vi "initialise.vi"(8 "error in (no error)":errorcluster, 11 "TrajectoryCN090716SpiralScan in":refnum<class "TrajectoryCN090716SpiralScan.lvclass">) -> (0 "error out":errorcluster, 3 "TrajectoryCN090716SpiralScan out":refnum<class "TrajectoryCN090716SpiralScan.lvclass">)   [LabVIEW 2010, in "TrajectoryCN090716SpiralScan.lvclass"]
uses:
  TrajectoryCN090716SpiralScan.lvclass
  <vilib>/Native 3D Graph/xcontrol/3DPC_SurfacePlot.xctl
  TrajectoryDL091126GenericVoxel/TrajectoryDL091126GenericVoxel/TrajectoryDL091126GenericVoxel.lvclass
  common/enumerations/functional_global_action_enum.ctl
  common/enumerations/x_y_z_enumeration.ctl
  TrajectoryCN090716SpiralScan.lvclass/TrajectoryCN090716SpiralScan.ctl
panel:
  out "z signal":dbl[](graph)
  out "3D Graph":refnum<class "Base Datatype.lvclass">[](xcontrol)
  out "x signal":dbl[](graph)
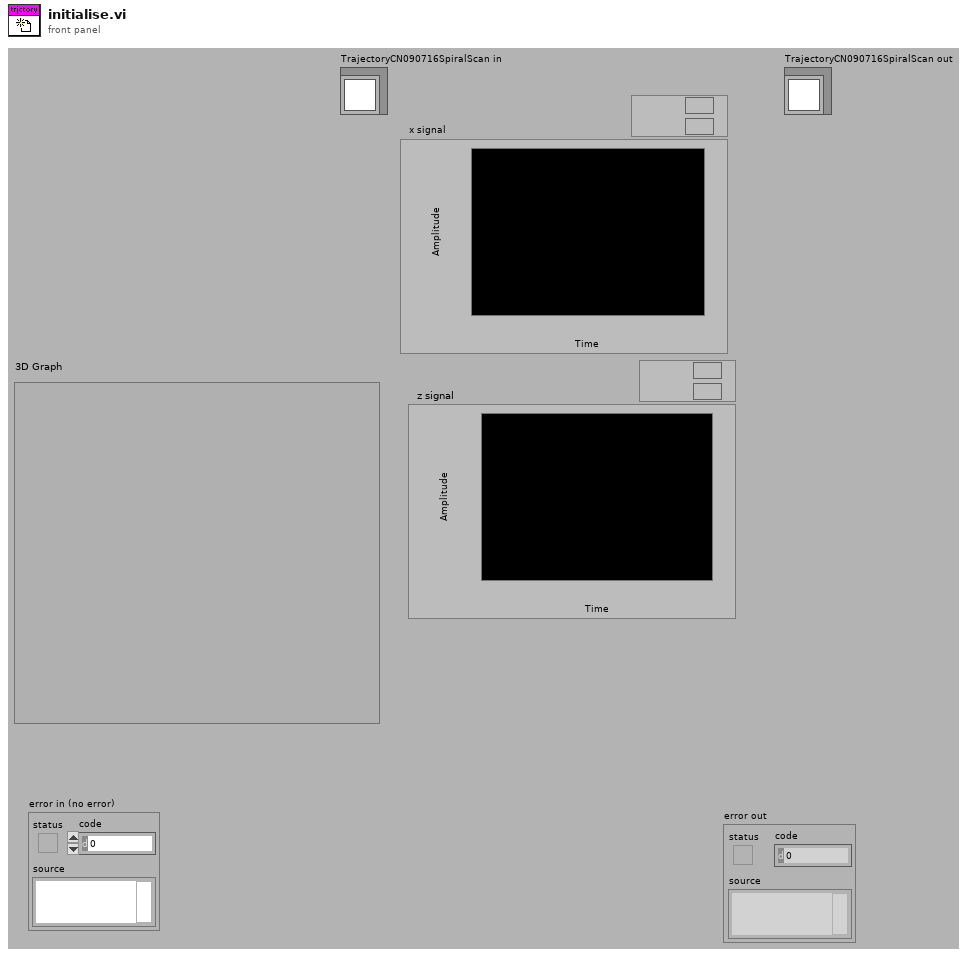
[diagram p1: front panel]
types:
  T1 = typedef "x_y_z_enumeration.ctl" = enum16{"x", "y", "z"}
  T2 = typedef "functional_global_action_enum.ctl" = enum16{"get", "set", "reset"}
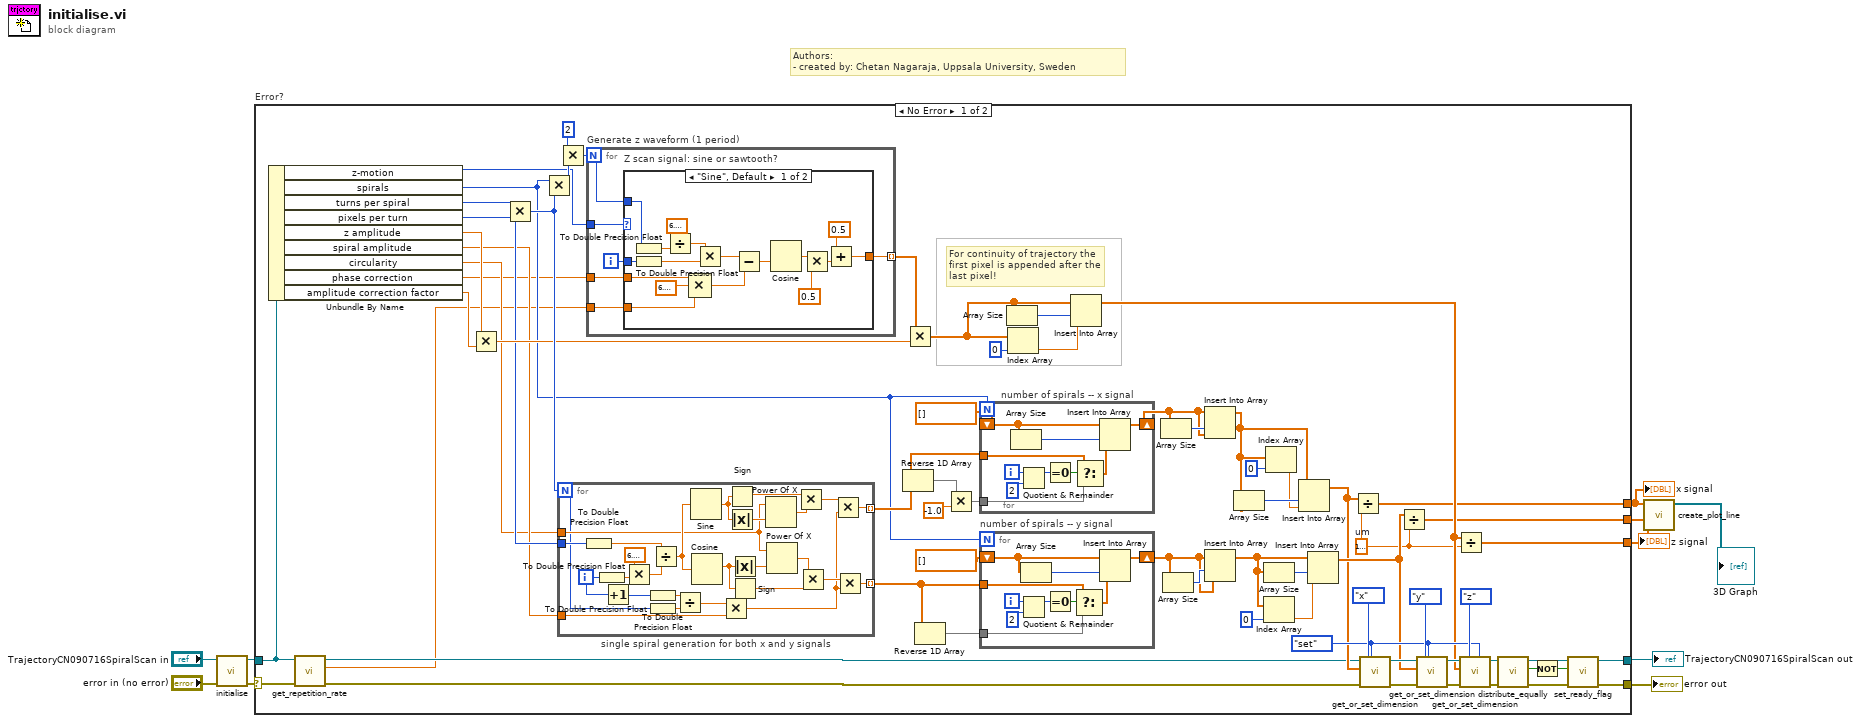
[diagram p0: block diagram]
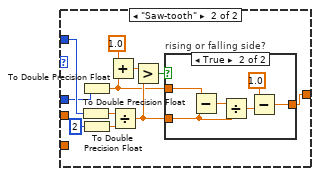
[diagram p2: hidden frame]
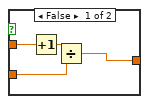
[diagram p3: hidden frame]
diagram:
  # "Authors: \n- created by: Chetan Nagaraja, Uppsala University, Sweden"
  n1 = call-parent "initialise.vi"("error in (no error)"="error in (no error)", "GenericTrajectory in"="TrajectoryCN090716SpiralScan in") -> ("error out"=w5:errorcluster, "GenericTrajectory out"=w6:refnum<class "TrajectoryCN090716SpiralScan.lvclass">)  [unwired: 8 out]
  n2 = case "Error?" shown="No Error" w5 {
    selector: w5 -> [w15 w169]
    tunnel: w6 -> [w13 w170]
    tunnel: [w33 w170] -> w10
    tunnel: [w30 w169] -> w9
    tunnel: [w39 _] -> w1
    tunnel: [w38 _] -> w3
    tunnel: [w29 _] -> w2
    frame No Error {
      w27 = dbl[unit] 1e-06  # um
      w70 = functional_global_action_enum."set" ("action")
      # "For continuity of trajectory the\nfirst pixel is appended after the \nlast pixel!"
      n3 = Unbundle By Name(w13) -> ("z-motion"=w22:enum16{"Sine", "Saw-tooth"}, "spirals"=w24:i32, "turns per spiral"=w23:i32, "pixels per turn"=w25:i32, "z amplitude"=w21:dbl[unit], "spiral amplitude"=w20:dbl[unit], "circularity"=w19:dbl, "phase correction"=w18:dbl[unit], "amplitude correction factor"=w17:dbl)
      n4 = call-dynamic "get_repetition_rate.vi"("error in (no error)"=w15, "GenericTrajectory in"=w13) -> ("error out"=w14:errorcluster, "repetition rate"=w11:dbl[unit], "GenericTrajectory out"=w12:refnum<class "TrajectoryCN090716SpiralScan.lvclass">)  [unwired: 7 in]
      n5 = Multiply(x=w21, y=w17) -> (x*y=w26:dbl[unit])
      n6 = Multiply(x=w23, y=w25) -> (x*y=w66:i32)
      n7 = Multiply(x=w24, y=w66) -> (x*y=w65:i32)
      n8 = Multiply(x=2, y=w65) -> (x*y=w59:i32)
      n9 = for "single spiral generation for both x and y signals" {
        N: w66 -> [w142]
        tunnel: w20 -> [w145]
        tunnel: [w156] -> w60 mode=indexing
        tunnel: [w155] -> w62 mode=indexing
        tunnel: w19 -> [w154]
        tunnel: w25 -> [w151]
        i -> [w146]
        n10 = To Double Precision Float(number=w151) -> (double precision float=w150:dbl)
        n11 = To Double Precision Float(number=w146) -> (double precision float=w152:dbl)
        n12 = Increment(x=w146) -> (x+1=w143:i32)
        n13 = Multiply(x=6.283185307179586, y=w152) -> (x*y=w153:dbl)
        n14 = To Double Precision Float(number=w143) -> (double precision float=w149:dbl)
        n15 = To Double Precision Float(number=w142) -> (double precision float=w148:dbl)
        n16 = Divide(x=w153, y=w150) -> (x/y=w160:dbl)
        n17 = Divide(x=w149, y=w148) -> (x/y=w147:dbl)
        n18 = Sine(x=w160) -> (sin(x)=w168:dbl)
        n19 = Cosine(x=w160) -> (cos(x)=w167:dbl)
        n20 = Multiply(x=w147, y=w145) -> (x*y=w144:dbl[unit])
        n21 = Sign(1:w168) -> (0:w164:dbl)
        n22 = Absolute Value(x=w168) -> (abs(x)=w165:dbl)
        n23 = Absolute Value(x=w167) -> (abs(x)=w166:dbl)
        n24 = Sign(1:w167) -> (0:w162:dbl)
        n25 = Power Of X(1:w165, 2:w154) -> (0:w163:dbl)
        n26 = Power Of X(1:w166, 2:w154) -> (0:w161:dbl)
        n27 = Multiply(x=w164, y=w163) -> (x*y=w158:dbl)
        n28 = Multiply(x=w161, y=w162) -> (x*y=w157:dbl)
        n29 = Multiply(x=w158, y=w144) -> (x*y=w156:dbl[unit])
        n30 = Multiply(x=w157, y=w144) -> (x*y=w155:dbl[unit])
      }
      n31 = for "Generate z waveform (1 period)" {
        N: w59 -> [w101]
        tunnel: w22 -> [w103]
        tunnel: [w102] -> w67 mode=indexing
        tunnel: w18 -> [w99]
        tunnel: w11 -> [w98]
        i -> [w100]
        n32 = case "Z scan signal: sine or sawtooth?" shown="\"Sine\", Default" w103 {
          tunnel: [w111 w129] -> w102
          tunnel: w101 -> [w118 w127]
          tunnel: w100 -> [w114 w123]
          tunnel: w99 -> [w107 _]
          tunnel: w98 -> [w105 _]
          frame "Sine", Default {
            n33 = To Double Precision Float(number=w118) -> (double precision float=w119:dbl)
            n34 = To Double Precision Float(number=w114) -> (double precision float=w113:dbl)
            n35 = Divide(x=6.283185307179586, y=w119) -> (x/y=w120:dbl)
            n36 = Compound Arithmetic op=MULTIPLY(w107, 6.283185307179586, w105) -> (w106:dbl)
            n37 = Multiply(x=w120, y=w113) -> (x*y=w109:dbl)
            n38 = Subtract(x=w109, y=w106) -> (x-y=w108:dbl)
            n39 = Cosine(x=w108) -> (cos(x)=w117:dbl)
            n40 = Multiply(x=w117, y=0.5) -> (x*y=w112:dbl)
            n41 = Add(x=0.5, y=w112) -> (x+y=w111:dbl)
          }
          frame "Saw-tooth" {
            n42 = To Double Precision Float(number=w127) -> (double precision float=w126:dbl)
            n43 = To Double Precision Float(number=w123) -> (double precision float=w121:dbl)
            n44 = To Double Precision Float(number=2 ("y")) -> (double precision float=w125:dbl)
            n45 = Add(x=1.0 ("y"), y=w121) -> (x+y=w124:dbl)
            n46 = Divide(x=w126, y=w125) -> (x/y=w130:dbl)
            n47 = Greater?(x=w124, y=w130) -> (0:w131:bool)
            n48 = case "rising or falling side?" shown="True" w131 {
              tunnel: w121 -> [w135 w141]
              tunnel: w130 -> [w133 w139]
              tunnel: [w132 w136] -> w129
              frame False {
                n49 = Increment(x=w135) -> (x+1=w134:dbl)
                n50 = Divide(x=w134, y=w133) -> (x/y=w132:dbl)
              }
              frame True {
                n51 = Subtract(x=w141, y=w139) -> (x-y=w140:dbl)
                n52 = Divide(x=w140, y=w139) -> (x/y=w138:dbl)
                n53 = Subtract(x=1.0, y=w138) -> (x-y=w136:dbl)
              }
            }
          }
        }
      }
      n54 = Reverse 1D Array(array=w60) -> (reversed array=w54:dbl[unit][])
      n55 = Multiply(x=w67, y=w26) -> (x*y=w16:dbl[unit][])
      n56 = Reverse 1D Array(array=w62) -> (reversed array=w56:dbl[unit][])
      n57 = Multiply(x=w54, y=-1.0) -> (x*y=w53:dbl[unit][])
      n58 = for "number of spirals -- x signal" {
        N: w24 -> [_]
        tunnel: w53 -> [w83]
        shift-right: [w80] -> w52
        shift-left: dbl[unit][] [] -> [w82]
        tunnel: w60 -> [w79]
        i -> [w87]
        n59 = Array Size(array=w82) -> (size(s)=w78:i32)
        n60 = Quotient & Remainder(x=w87, y=2) -> (x-y*floor(x/y)=w85:i32)  [unwired: 1 out]
        n61 = Equal To 0?(x=w85) -> (x = 0?=w84:bool)
        n62 = Select(t=w79, s=w84, f=w83) -> (s? t:f=w81:dbl[unit][])
        n63 = Insert Into Array(array=w82, index=w78, new element=w81) -> (w80:dbl[unit][])
      }
      n64 = for "number of spirals -- y signal" {
        N: w24 -> [_]
        tunnel: w56 -> [w93]
        shift-right: [w90] -> w47
        shift-left: dbl[unit][] [] -> [w92]
        tunnel: w62 -> [w89]
        i -> [w97]
        n65 = Quotient & Remainder(x=w97, y=2) -> (x-y*floor(x/y)=w95:i32)  [unwired: 1 out]
        n66 = Array Size(array=w92) -> (size(s)=w88:i32)
        n67 = Equal To 0?(x=w95) -> (x = 0?=w94:bool)
        n68 = Select(t=w89, s=w94, f=w93) -> (s? t:f=w91:dbl[unit][])
        n69 = Insert Into Array(array=w92, index=w88, new element=w91) -> (w90:dbl[unit][])
      }
      n70 = Array Size(array=w16) -> (size(s)=w43:i32)
      n71 = Index Array(array=w16, index=0) -> (element=w42:dbl[unit])
      n72 = Insert Into Array(array=w16, index=w43, new element=w42) -> (w40:dbl[unit][])
      n73 = Array Size(array=w52) -> (size(s)=w58:i32)
      n74 = Array Size(array=w47) -> (size(s)=w57:i32)
      n75 = Insert Into Array(array=w52, index=w58, new element=w52) -> (w48:dbl[unit][])
      n76 = Insert Into Array(array=w47, index=w57, new element=w47) -> (w45:dbl[unit][])
      n77 = Array Size(array=w48) -> (size(s)=w51:i32)
      n78 = Array Size(array=w45) -> (size(s)=w44:i32)
      n79 = Index Array(array=w45, index=0) -> (element=w46:dbl[unit])
      n80 = Index Array(array=w48, index=0) -> (element=w50:dbl[unit])
      n81 = Insert Into Array(array=w48, index=w51, new element=w50) -> (w28:dbl[unit][])
      n82 = Insert Into Array(array=w45, index=w44, new element=w46) -> (w36:dbl[unit][])
      n83 = Divide(x=w28, y=w27) -> (x/y=w39:dbl[])
      n84 = call-dynamic "get_or_set_dimension.vi"("dimension"=x_y_z_enumeration."x", "action"=w70, "error in (no error)"=w14, "pixel values in (single dimension)"=w28, "GenericTrajectory in"=w12) -> ("error out"=w76:errorcluster, "GenericTrajectory out"=w75:refnum<class "TrajectoryCN090716SpiralScan.lvclass">)  [unwired: 1 in, 4 out]
      n85 = Divide(x=w36, y=w27) -> (x/y=w38:dbl[])
      n86 = call-dynamic "get_or_set_dimension.vi"("dimension"=x_y_z_enumeration."y", "action"=w70, "error in (no error)"=w76, "pixel values in (single dimension)"=w36, "GenericTrajectory in"=w75) -> ("error out"=w73:errorcluster, "GenericTrajectory out"=w72:refnum<class "TrajectoryCN090716SpiralScan.lvclass">)  [unwired: 1 in, 4 out]
      n87 = Divide(x=w40, y=w27) -> (x/y=w29:dbl[])
      n88 = call-dynamic "get_or_set_dimension.vi"("dimension"=x_y_z_enumeration."z", "action"=w70, "error in (no error)"=w73, "pixel values in (single dimension)"=w40, "GenericTrajectory in"=w72) -> ("error out"=w69:errorcluster, "GenericTrajectory out"=w68:refnum<class "TrajectoryCN090716SpiralScan.lvclass">)  [unwired: 1 in, 4 out]
      n89 = call-dynamic "distribute_equally.vi"("error in (no error)"=w69, "TrajectoryDL091126GenericVoxel in"=w68) -> ("error out"=w31:errorcluster, "failed?"=w35:bool, "TrajectoryDL091126GenericVoxel out"=w34:refnum<class "TrajectoryCN090716SpiralScan.lvclass">)  [unwired: 7 in]
      n90 = Not(x=w35) -> (.not. x?=w32:bool)
      n91 = call-dynamic "set_ready_flag.vi"("error in (no error)"=w31, "ready for initialisation?"=w32, "GenericTrajectory in"=w34) -> ("error out"=w30:errorcluster, "GenericTrajectory out"=w33:refnum<class "TrajectoryCN090716SpiralScan.lvclass">)  [unwired: 7 in]
    }
    frame Error {
    }
  }
  "error out" <- w9
  "TrajectoryCN090716SpiralScan out" <- w10
  "x signal" <- w1
  "z signal" <- w2
  n92 = call <vilib>:"create_plot_line.vi"("z vector"=w2, "y vector"=w3, "x vector"=w1) -> ("plots out"=→"3D Graph":refnum<class "Base Datatype.lvclass">[])  [unwired: 2 in, 6 out]
